vi "Engine - Generic - VVA Host.vi"() -> ()   [LabVIEW 2015, in "ECS-Host.lvlib"]
uses:
  ECS-Host.lvlib
panel:
  out "Cam2AdvStp":sgl caption="[CAD]" format="%#.2f"
  out "Cam1AdvStp":sgl caption="[CAD]" format="%#.2f"
  out "Cam1_KpOut":sgl(slide) caption="IMV  Kc Action" max=0 scale=0.0..1.0 scale format="%#.2f"
  out "Cam1_TiOut":sgl(slide) caption="IMV  Ti Action" max=0 scale=0.0..100.0 scale format="%#.2f"
  out "Cam1_TdOut":sgl(slide) caption="IMV  Td Action" max=0 scale=0.0..100.0 scale format="%#.2f"
  out "Cam1_PIDOut":sgl caption="[]" format="%#.2f"
  in  "Cam1_PIDE":bool caption="Cam1 PIDEnable"
  in  "Cam1_PIDMax":sgl caption="[]" format="%#.2f"
  in  "Cam1_PIDMin":sgl caption="[]" format="%#.2f"
  in  "Cam1NomResistance":sgl caption="[W]" format="%#.2f"
  in  "Cam1_Ti":sgl caption="[]" format="%#.3f"
  in  "Cam1_Td":sgl caption="[]" format="%#.3f"
  in  "Cam1_PIDFF":sgl caption="[]" format="%#.2f"
  in  "Cam1_Kp":sgl caption="[%/CAD]" format="%#.3f"
  out "Cam2_KpOut":sgl(slide) caption="IMV  Kc Action" max=0 scale=0.0..1.0 scale format="%#.2f"
  out "Cam2_TiOut":sgl(slide) caption="IMV  Ti Action" max=0 scale=0.0..100.0 scale format="%#.2f"
  out "Cam2_TdOut":sgl(slide) caption="IMV  Td Action" max=0 scale=0.0..100.0 scale format="%#.2f"
  out "Cam2_PIDOut":sgl caption="[]" format="%#.2f"
  in  "Cam2_PIDE":bool caption="Cam1 PIDEnable"
  in  "Cam2_PIDMax":sgl caption="[]" format="%#.2f"
  in  "Cam2_PIDMin":sgl caption="[]" format="%#.2f"
  in  "Cam2NomResistance":sgl caption="[W]" format="%#.2f"
  in  "Cam2_Ti":sgl caption="[]" format="%#.3f"
  in  "Cam2_Td":sgl caption="[]" format="%#.3f"
  in  "Cam2_PIDFF":sgl caption="[]" format="%#.2f"
  in  "Cam2_Kp":sgl caption="[%/CAD]" format="%#.3f"
  out "Cam2DutyCyc_Des":sgl caption="[%]" format="%#.2f"
  out "Cam2DutyCyc_MaxCalc":sgl caption="[]" format="%#.2f"
  out "Cam2Current_Calc":sgl caption="[]" format="%#.2f"
  in  "Cam2Ctrl_E":bool caption="Cam1 ControlEnable"
  in  "Cam2DutyCyc_ManE":bool caption="Cam1 ManualOverride"
  in  "Cam2DutyCyc_Min":sgl caption="[]" format="%#.2f"
  in  "Cam2DutyCyc_Man":sgl caption="[%]" format="%#.2f"
  in  "Cam2PWMFreq":sgl caption="[Hz]" format="%#.2f"
  in  "Cam2DutyCyc_Max":sgl caption="[]" format="%#.2f"
  in  "Cam2_NonPIDFF":sgl caption="[]" format="%#.2f"
  out "Cam1DutyCyc_Des":sgl caption="[%]" format="%#.2f"
  out "Cam1DutyCyc_MaxCalc":sgl caption="[]" format="%#.2f"
  out "Cam1Current_Calc":sgl caption="[]" format="%#.2f"
  in  "Cam1Ctrl_E":bool caption="Cam1 ControlEnable"
  in  "Cam1DutyCyc_ManE":bool caption="Cam1 ManualOverride"
  in  "Cam1DutyCyc_Min":sgl caption="[]" format="%#.2f"
  in  "Cam1DutyCyc_Man":sgl caption="[%]" format="%#.2f"
  in  "Cam1PWMFreq":sgl caption="[Hz]" format="%#.2f"
  in  "Cam1DutyCyc_Max":sgl caption="[]" format="%#.2f"
  in  "Cam1_NonPIDFF":sgl caption="[]" format="%#.2f"
  # "+"
  # "+"
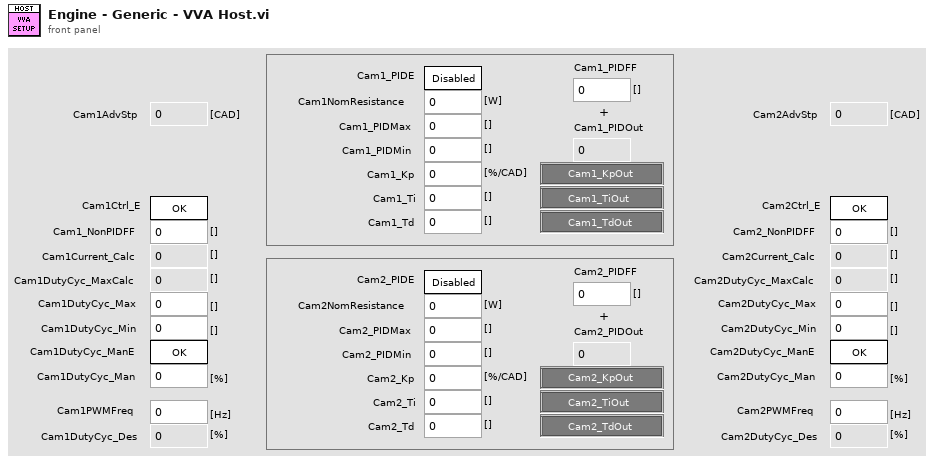
[diagram p1: front panel]
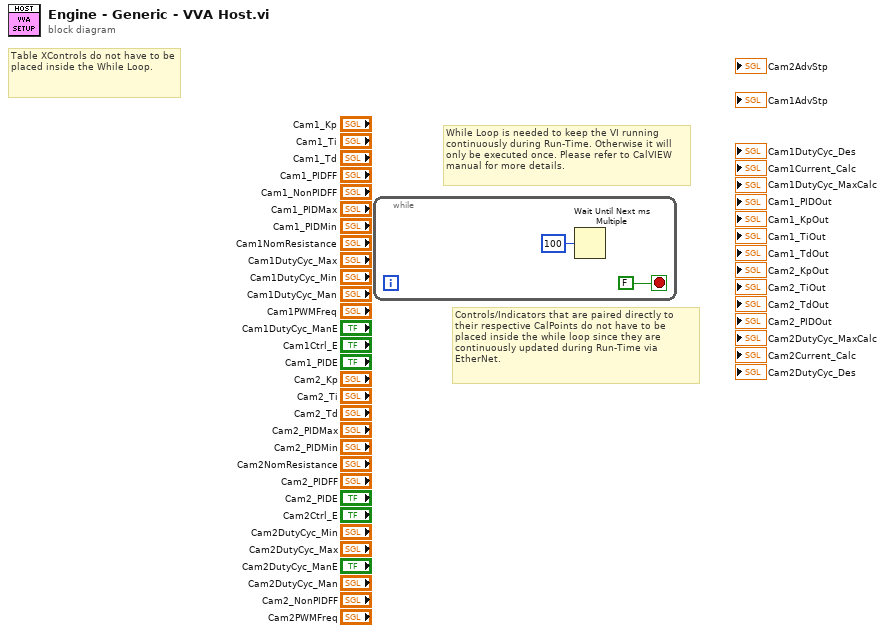
[diagram p0: block diagram]
diagram:
  # "Table XControls do not have to be placed inside the While Loop."
  # "Controls/Indicators that are paired directly to their respective CalPoints do not have to be placed inside the while loop since they are continuously updated during Run-Time via EtherNet."
  # "While Loop is needed to keep the VI running\ncontinuously during Run-Time. Otherwise it will only be executed once. Please refer to CalVIEW manual for more details."
  n1 = while {
    stop <- FALSE ("Stop Button") stop-if-true
    n2 = Wait Until Next ms Multiple(millisecond multiple=u32 100) -> ()  [unwired: 1 out]
  }
